vi "ZLIB Get Global Info__ogtk.vi"(4 "error in (no error)":errorcluster, 7 "unzip Refnum":T1) -> (0 "error out":errorcluster, 1 "nEntry":u32, 2 "global comment":string, 3 "unzip Refnum out":T1)   [LabVIEW 2012]
doc: "Gets the global info of an archive in an unzip session."
uses:
  <userlib>/_OpenG.lib/lvzip/lvzip.llb/ZLIB Unzip Handle__ogtk.ctl
  <userlib>/_OpenG.lib/lvzip/lvzlib.dll
panel:
  # "Please visit http://www.OpenG.org to learn about the\nOpen Source LabVIEW software movement.\n\nNOTICE -- YOU MUST LEAVE THIS NOTICE IN PLACE.  PER THE TERMS OF THE LICENSE BELOW, YOU MAY SUBLICENSE THIS SOFTWARE \nIN ANY WAY THAT DOES NOT CONFLICT WITH THIS LICENSE.\n\n### BSD License (http://www.opensource.org/licenses/bsd-license.php) Begin ###\n \nCopyright (C) 2002 Rolf Kalbermatter rolf.kalbermatter@citeng.com\nCopyright (C) 2002 Jim Kring jim@jimkring.com\n\nAll rights reserved.\n\nRedistribution and use in source and binary forms, with or without modification, are permitted provided that the following conditions are met:\n\n    * Redistributions of source code must retain the above copyright notice, this list of conditions and the following disclaimer.\n    * Redistributions in binary form must reproduce the above copyright notice, this list of conditions and the following disclaimer in the \n       documentation and/or other materials provided with the distribution.\n    * Neither the name of SciWare, James Kring, Inc., nor the names of its contributors may be used to endorse or promote products derived \n       from this software without specific prior written permission.\n\nTHIS SOFTWARE IS PROVIDED BY THE COPYRIGHT HOLDERS AND CONTRIBUTORS \"AS IS\" AND ANY EXPRESS OR IMPLIED WARRANTIES, \nINCLUDING, BUT NOT LIMITED TO, THE IMPLIED WARRANTIES OF MERCHANTABILITY AND FITNESS FOR A PARTICULAR PURPOSE ARE \nDISCLAIMED. IN NO EVENT SHALL THE COPYRIGHT OWNER OR CONTRIBUTORS BE LIABLE FOR ANY DIRECT, INDIRECT, INCIDENTAL,\n SPECIAL, EXEMPLARY, OR CONSEQUENTIAL DAMAGES (INCLUDING, BUT NOT LIMITED TO, PROCUREMENT OF SUBSTITUTE GOODS OR \nSERVICES; LOSS OF USE, DATA, OR PROFITS; OR BUSINESS INTERRUPTION) HOWEVER CAUSED AND ON ANY THEORY OF LIABILITY, \nWHETHER IN CONTRACT, STRICT LIABILITY, OR TORT (INCLUDING NEGLIGENCE OR OTHERWISE) ARISING IN ANY WAY OUT OF THE USE \nOF THIS SOFTWARE, EVEN IF ADVISED OF THE POSSIBILITY OF SUCH DAMAGE.\n\n### BSD License End ###"
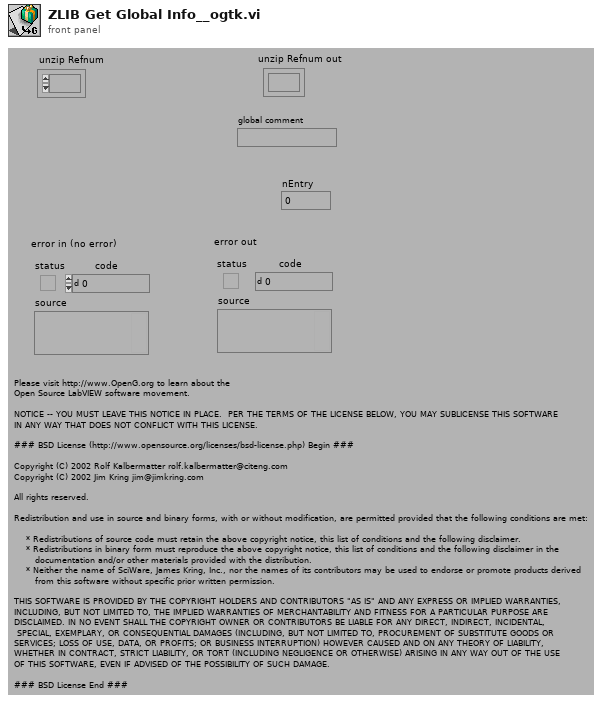
[diagram p1: front panel]
types:
  T1 = typedef "ZLIB Unzip Handle__ogtk.ctl" = refnum<k1>
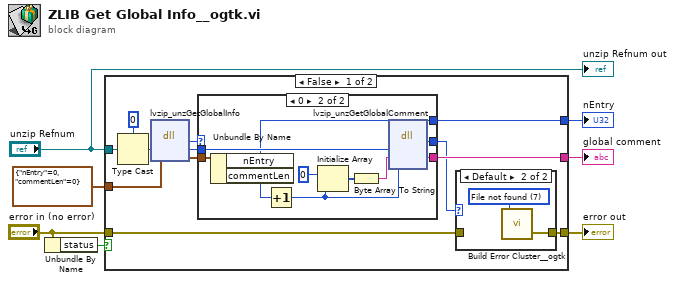
[diagram p0: block diagram]
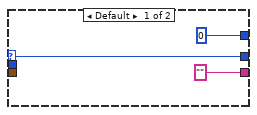
[diagram p3: hidden frame]
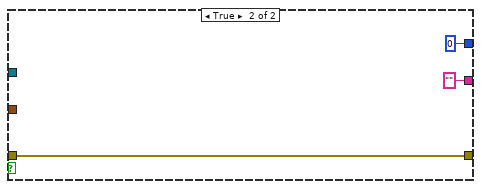
[diagram p4: hidden frame]
diagram:
  n1 = Unbundle By Name("error in (no error)") -> ("status"=w7:bool)
  n2 = case shown="False" w7 {
    tunnel: "error in (no error)" -> [w9 w38]
    tunnel: [w18 w38] -> w4
    tunnel: "unzip Refnum" -> [w16 _]
    tunnel: cluster{"nEntry":u32, "commentLen":u32} {"nEntry"=0, "commentLen"=0} -> [w13 _]
    tunnel: [w11 "" ("comment")] -> w2
    tunnel: [w10 u32 0 ("nEntry")] -> w1
    frame False {
      n3 = Type Cast(type=u32 0 ("unzFile"), x=w16) -> (*(type *) &x=w15:u32)
      n4 = dll-call lib="C:/Program Files/National Instruments/LabVIEW 2012/user.lib/_OpenG.lib/lvzip/lvzlib.*" fn="lvzip_unzGetGlobalInfo"("unzFile"=w15, w13) -> (w19:i32, "unzFile"=w14:u32, w12:cluster{"nEntry":u32, "commentLen":u32})  [unwired: 3 in, 2 out]
      n5 = case shown="0" w19 {
        selector: w19 -> [w23 _]
        tunnel: w14 -> [_ w34]
        tunnel: w12 -> [_ w35]
        tunnel: ["" ("comment") w28] -> w11
        tunnel: [u32 0 ("nEntry") w26] -> w10
        tunnel: [w23 w27] -> w8
        frame Default {
        }
        frame 0 {
          n6 = Unbundle By Name(w35) -> ("nEntry"=w26:u32, "commentLen"=w32:u32)
          n7 = Increment(x=w32) -> (x+1=w29:u32)
          n8 = Initialize Array(u8 0 ("Element Data"), w29) -> (w33:u8[])
          n9 = Byte Array To String(unsigned byte array=w33) -> (string=w30:string)
          n10 = dll-call lib="C:/Program Files/National Instruments/LabVIEW 2012/user.lib/_OpenG.lib/lvzip/lvzlib.*" fn="lvzip_unzGetGlobalComment"("unzFile"=w34, "comment"=w30, "commentLen"=w29) -> (w27:i32, "comment"=w28:string)  [unwired: 5 in, 2 out]
        }
      }
      n11 = case shown="Default" w8 {
        tunnel: w9 -> [w20 _]
        tunnel: [w20 w21] -> w18
        frame 0.. {
        }
        frame Default {
          w22 = 7 items=["No error", "Argument error", "Memory is full", "Out of zone", "End of file", "File already open", "Generic file I/O error", "File not found", "File permission error", "Disk is full", "Duplicate path", "Too many files open", "System feature not enabled", "Resource file not found", "Cannot add resource", "Resource not found", "Image not found", "Image memory error", "Pen does not exist", "Config type invalid", "Config token not found", "Config parse error", "Config memory error", "Bad external code format", "Bad external code offset", "External code not present", "Null window", "Destroy window error", "Null menu", "Print aborted", "Bad print record", "Print driver error", "Windows error during printing", "Memory error during printing", "Print dialog error", "Generic print error", "Invalid device refnum", "Device not found", "Device parameter error", "Device unit error", "Cannot open device", "Device call aborted", "Generic error", "Cancelled by user", "Object ID too low", "Object ID too high", "Object not in heap", "Unknown heap", "Unknown object (invalid DefProc)", "Unknown object (DefProc not in table)", "Message out of range", "Invalid (null) method", "Unknown message", "Manager call not supported", "Bad address", "Network operation in progress", "Network operation timed out", "Connection is busy", "Network attribute not supported", "Network error", "Address in use", "System out of memory", "Connection aborted", "Connection refused", "Not connected", "Already connected", "Connection closed", "Initialization error (interapplication manager)", "Bad occurrence", "Wait on unbound occurrence handler", "Occurrence queue overflow", "Datalog type conflict", "Unused", "Unrecognized type (interapplication manager)", "Memory corrupt", "Failed to make temporary DLL", "Old CIN version", "Drag socket not found", "Failed to load drop-object", "Failed to register OLE object", "Failed to release OLE object", "Format specifier type mismatch", "Unknown format specifier", "Too few format specifiers", "Too many format specifiers", "Scan failed", "Newer CIN version", "Error converting to variant", "Runtime menu error", "Password tampered", "Variant attribute not found", "Incompatible variant data type", "Event data is not available", "Event Store is not present", "Occurrence is not found", "Event Queue is not created", "Event info is not available", "Refnum passed is NULL", "Error retrieving Class GUID", "Error retrieving CoClass GUID", "Error retrieving TypeLib GUID.", "Bad built application magic bytes.", "Specific driver is different from the specific driver associated with the Logical Name.", "There is no session opened to the class driver.", "Max Error", "MAX - Error with config objects", "MAX - Error loading configuration", "MAX - Group not supported"]
          n12 = call <userlib>:"Build Error Cluster__ogtk.vi"("code"=w22) -> ("error out"=w21:errorcluster)  [unwired: 1 in]
        }
      }
    }
    frame True {
    }
  }
  "error out" <- w4
  "global comment" <- w2
  "nEntry" <- w1
  "unzip Refnum out" <- "unzip Refnum"
